vi "Pre Launch Init.vi"(11 "AE75TX in":refnum<class "AE75TX.lvclass">) -> (0 "error out":errorcluster, 3 "AE75TX out":refnum<class "AE75TX.lvclass">)   [LabVIEW 2015, in "AE75TX Actor.lvlib" / "AE75TX.lvclass"]
doc: "(<B>Filename</B>: Actor Framework.lvlib:Actor.lvclass:Pre Launch Init.vi)\n\nDefines behavior that occurs after the Launch Nested Actor method is invoked but before the actor's Actor Core method begins running.\n\nBy default, this method does nothing. A descendant class may override it to define behavior."
uses:
  AE75TX.lvclass
  AE75TX.lvclass/AE75TX.ctl
  Controls/PV Full Data Cluster.ctl
  Controls/PV Standard Value Cluster.ctl
  <vilib>/ActorFramework/Actor/Actor.lvclass
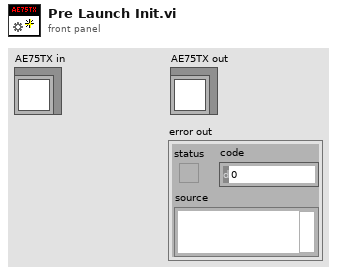
[diagram p1: front panel]
types:
  T1 = typedef "AE75TX Actor.lvlib/AE75TX.lvclass/PV Full Data Cluster.ctl" = cluster{"PV Standard Values":T2, "Reactive Power (kVAR)":sgl}
  T2 = typedef "AE75TX Actor.lvlib/AE75TX.lvclass/PV Standard Value Cluster.ctl" = cluster{"Va (V)":sgl, "Vb (V)":sgl, "Vc (V)":sgl, "Ia (A)":sgl, "Ib (A)":sgl, "Ic (A)":sgl, "Vdc (V)":sgl, "Idc (A)":sgl, "Frequency (Hz)":sgl, "Line Power (kW)":sgl, "Total Power (kWh)":u32, "PV Input (V)":sgl, "DC Power (kW)":sgl}
  T3 = typedef "AE75TX Actor.lvlib/AE75TX.lvclass/AE75TX Notifiers.ctl" = cluster{"stop":refnum<notifier>, "data":refnum<notifier>}
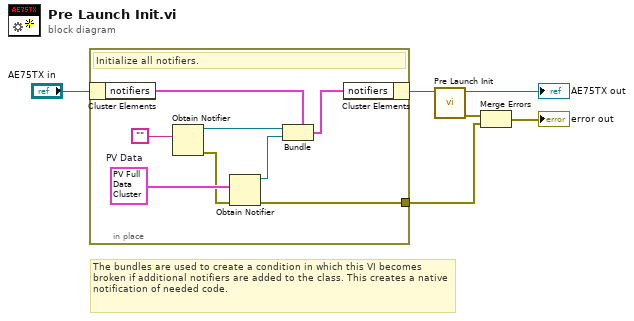
[diagram p0: block diagram]
diagram:
  # "The bundles are used to create a condition in which this VI becomes broken if additional notifiers are added to the class. This creates a native notification of needed code."
  n1 = in-place {
    in-place-border: [w7] -> w1
    w14 = T1 {"PV Standard Values"={"Va (V)"=0.0, "Vb (V)"=0.0, "Vc (V)"=0.0, "Ia (A)"=0.0, "Ib (A)"=0.0, "Ic (A)"=0.0, "Vdc (V)"=0.0, "Idc (A)"=0.0, "Frequency (Hz)"=0.0, "Line Power (kW)"=0.0, "Total Power (kWh)"=0, "PV Input (V)"=0.0, "DC Power (kW)"=0.0}, "Reactive Power (kVAR)"=0.0}  # PV Data
    # "Initialize all notifiers."
    n2 = in-place-cluster #1("AE75TX in") -> ("notifiers"=w11:T3)
    n3 = Obtain Notifier(notification data type="") -> (notifier out=w12:refnum<notifier>, error out=w8:errorcluster)  [unwired: 3 in, 1 out]
    n4 = Obtain Notifier(notification data type=w14, error in (no error)=w8) -> (notifier out=w9:refnum<notifier>, error out=w7:errorcluster)  [unwired: 2 in, 1 out]
    n5 = Bundle(cluster=w11, "stop"=w12, "data"=w9) -> (w10:T3)
    n6 = in-place-cluster #1("notifiers"=w10) -> (w4:refnum<class "AE75TX.lvclass">)
  }
  n7 = call-parent "Pre Launch Init.vi"("Actor in"=w4) -> ("error out"=w6:errorcluster, "Actor out"=→"AE75TX out":refnum<class "AE75TX.lvclass">)  [unwired: 9 in]
  n8 = Merge Errors(w6, w1) -> (→"error out":errorcluster)
